vi "Energy to Pull-back_linear_subVI.vi"(11 "Puck Energy Requirement (mJ)":dbl) -> (1 "Output Velocity":dbl, 2 "Pull-back angle (rad)":dbl, 3 "Pull-back angle (°)":dbl)   [LabVIEW 2017]
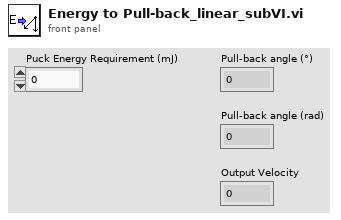
[diagram p1: front panel]
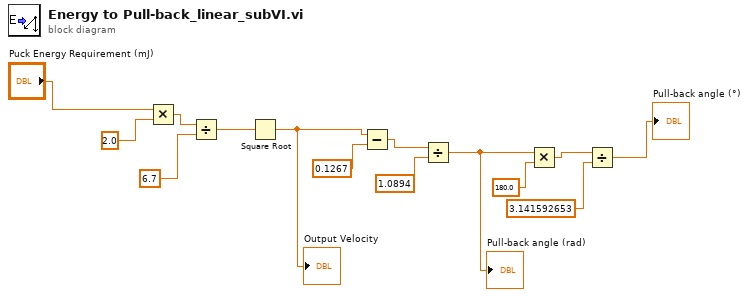
[diagram p0: block diagram]
diagram:
  n1 = Multiply(x="Puck Energy Requirement (mJ)", y=2.0) -> (x*y=w4:dbl)
  n2 = Divide(x=w4, y=6.7) -> (x/y=w1:dbl)
  n3 = Square Root(x=w1) -> (sqrt(x)=w6:dbl)
  "Output Velocity" <- w6
  n4 = Subtract(x=w6, y=0.1267) -> (x-y=w8:dbl)
  n5 = Divide(x=w8, y=1.0894) -> (x/y=w10:dbl)
  "Pull-back angle (rad)" <- w10
  n6 = Multiply(x=w10, y=180.0) -> (x*y=w13:dbl)
  n7 = Divide(x=w13, y=3.141592653) -> (x/y=→"Pull-back angle (°)":dbl)
